vi "Begin.vi"(8 "error in":errorcluster) -> (0 "error out":errorcluster)   [LabVIEW 2020]
doc: "Called before other user functions, this VI is expected to open initial I/O refnums, load in file data, and do all program initialization. Notice that the <B>error out</B> terminal is simply used for data flow. Wiring it to other structures or subVIs ensures that this VI runs first."
uses:
  <vilib>/Rock Robotics/WPI/SafetyOutput/WPI_SafetyOutputConfigMenu.ctl
  <vilib>/Rock Robotics/WPI/DriverStation/WPI_DriverStationRobotMode2.ctl
  <vilib>/Rock Robotics/WPI/ThirdParty/REV Robotics/REVLib/Typedef/Spark MAX Motor Type.ctl
  <vilib>/Rock Robotics/WPI/ThirdParty/REV Robotics/REVLib/Typedef/Spark MAX Idle Mode.ctl
  <vilib>/Rock Robotics/WPI/ThirdParty/Phoenix-LabVIEW/Motor Controller/Controls/CTRE_Phoenix_MotorControl_ControlMode.ctl
  <vilib>/Rock Robotics/WPI/Joystick/WPI_JoystickDeviceEnum.ctl
  <vilib>/Rock Robotics/WPI/Solenoid/WPI_SolenoidChannel.ctl
  <vilib>/Rock Robotics/SystemInterfaces/i2clib/i2c_bus.ctl
  <vilib>/Rock Robotics/WPI/DriverStation/WPI_DriverStationAllianceInfo.ctl
  Robot Global Data.vi
  <vilib>/Rock Robotics/Network Tables/NT Write String Array.vi
  <vilib>/Rock Robotics/WPI/RobotDrive/WPI_RobotDriveOpen2MotorWithExistingMotors.vi
  <vilib>/Rock Robotics/WPI/Solenoid/WPI_SolenoidOpenDouble.vi
  Global Variables/StateMachineOperation.vi
panel:
  in  "Nothing":cluster{"R":dbl, "G":dbl, "B":dbl}={"R"=0.143, "G"=0.427, "B"=0.429}
  in  "Red Calibration":cluster{"R":dbl, "G":dbl, "B":dbl}={"R"=0.525, "G"=0.346, "B"=0.128}
  in  "Blue Calibration":cluster{"R":dbl, "G":dbl, "B":dbl}={"R"=0.143, "G"=0.427, "B"=0.429}
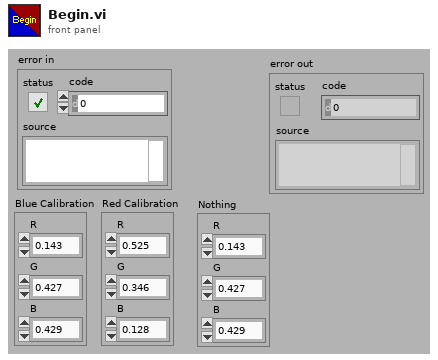
[diagram p1: front panel]
types:
  T1 = typedef "WPI_SolenoidChannel.ctl" = enum8{"Solenoid 0", "Solenoid 1", "Solenoid 2", "Solenoid 3", "Solenoid 4", "Solenoid 5", "Solenoid 6", "Solenoid 7", "Solenoid 8", "Solenoid 9", "Solenoid 10", "Solenoid 11", "Solenoid 12", "Solenoid 13", "Solenoid 14", "Solenoid 15", "Invalid"}
  T2 = typedef "WPI_DriverStationAllianceInfo.ctl" = enum16{"Red", "Blue", "Invalid"}
  T3 = typedef "i2c_bus.ctl" = enum16{"I2C On-Board", "I2C MXP", "Invalid"}
  T4 = typedef "WPI_JoystickDeviceEnum.ctl" = enum16{"USB 0", "USB 1", "USB 2", "USB 3", "USB 4", "USB 5"}
  T5 = typedef "CTRE_Phoenix_MotorControl_ControlMode.ctl" = u16
  T6 = typedef "Spark MAX Idle Mode.ctl" = enum16{"Coast", "Brake"}
  T7 = typedef "Spark MAX Motor Type.ctl" = enum16{"Brushed", "Brushless"}
  T8 = typedef "WPI_DriverStationRobotMode2.ctl" = enum16{"Autonomous Disabled", "Autonomous Enabled", "Teleop Disabled", "Teleop Enabled", "Disconnected", "Finish", "Test Disabled", "Test Enabled", "Emergency Stopped"}
  T9 = typedef "WPI_SafetyOutputConfigMenu.ctl" = enum16{"Enable", "Disable"}
  T10 = typedef "WPI_MotorControlDeviceRef.ctl" = cluster{"DeviceStatus":errorcluster, "Type":T11, "PWM":cluster{"PWM Channel":T12, "DeadBand":T13}, "CAN":cluster{"Device Number":u8, "SetOutput VI Ref":variant, "GetOutput VI Ref":variant, "Enable VI Ref":variant, "Disable VI Ref":variant, "Data":variant}, "Invert":bool, "DIO PWM":cluster{"PWM \"Enable\" Channel":T12, "DIOChannel":T14, "PWM Rate":dbl}}
  T11 = typedef "WPI_MotorControlType.ctl" = enum16{"PWM", "CAN", "DIO PWM"}
  T12 = typedef "FPGA_DIOPWMChannel.ctl" = enum8{"PWM 0", "PWM 1", "PWM 2", "PWM 3", "PWM 4", "PWM 5", "PWM 6", "PWM 7", "PWM 8", "PWM 9", "PWM MXP 0", "PWM MXP 1", "PWM MXP 2", "PWM MXP 3", "PWM MXP 4", "PWM MXP 5", "PWM MXP 6", "PWM MXP 7", "PWM MXP 8", "PWM MXP 9", "Invalid"}
  T13 = typedef "WPI_PWMDeadband.ctl" = cluster{"Name":string, "maxPositivePwm":i32, "minPositivePwm":i32, "centerPwm":i32, "maxNegativePwm":i32, "minNegativePwm":i32, "angularRange":u16}
  T14 = typedef "FPGA_DIOChannel.ctl" = enum8{"DIO 0", "DIO 1", "DIO 2", "DIO 3", "DIO 4", "DIO 5", "DIO 6", "DIO 7", "DIO 8", "DIO 9", "DIO MXP 0", "DIO MXP 1", "DIO MXP 2", "DIO MXP 3", "DIO MXP 4", "DIO MXP 5", "DIO MXP 6", "DIO MXP 7", "DIO MXP 8", "DIO MXP 9", "DIO MXP 10", "DIO MXP 11", "DIO MXP 12", "DIO MXP 13", "DIO MXP 14", "DIO MXP 15", "SPI Port CS1", "SPI Port CS2", "SPI Port CS3", "SPI Port MISO", "SPI Port MOSI", "Invalid"}
  T15 = typedef "WPI_JoystickDevRef.ctl" = cluster{"Device":T4}
  T16 = typedef "WPI_RobotDriveDevRef.ctl" = cluster{"DevStatus":errorcluster, "Motors[]":T10[], "Square Inputs":bool, "Max Output":dbl}
  T17 = typedef "WPI_SolenoidDevRef.ctl" = cluster{"DevStatus":errorcluster, "Pneumatics Control Module":u8, "Forward Solenoid Channel":T1, "Reverse Solenoid Channel":T1}
  T18 = typedef "Color Sensor V3 DevRef.ctl" = cluster{"I2CDevRef":T19}
  T19 = typedef "WPI_I2CDevRef.ctl" = cluster{"DevStatus":errorcluster, "Device Address":u8, "Handle":i32, "I2C Bus":T3}
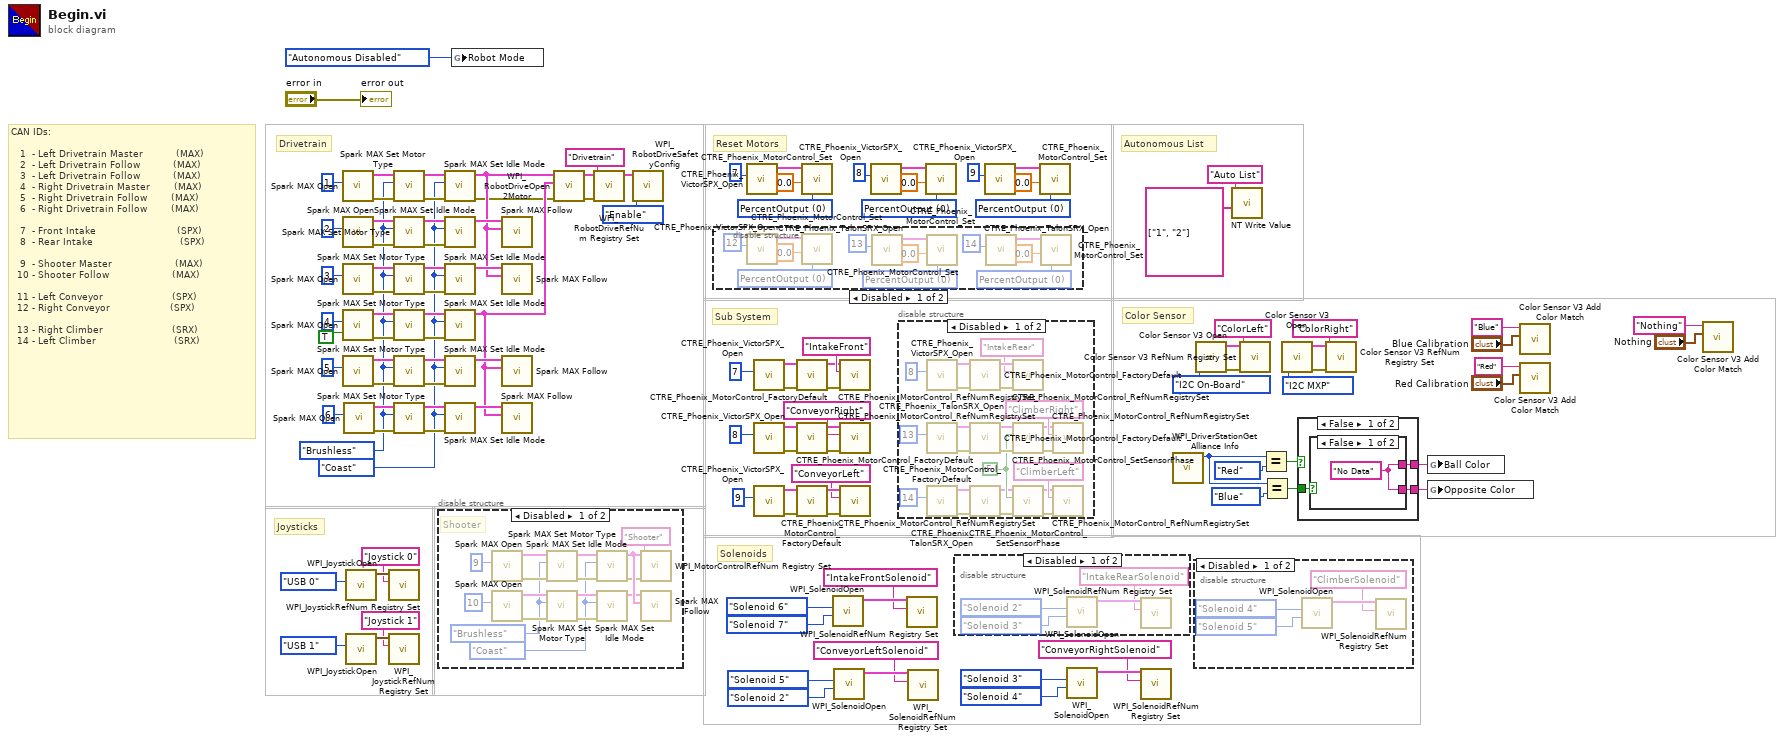
[diagram p0: block diagram]
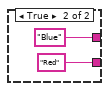
[diagram p6: hidden frame]
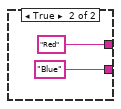
[diagram p7: hidden frame]
diagram:
  w59 = T5 0 items=["PercentOutput"=0, "Position"=1, "Velocity"=2, "Current"=3, "Follower"=5, "MotionProfile"=6, "MotionMagic"=7, "MotionProfileArc"=10, "Disabled"=15] ("Control Mode")
  w64 = T5 0 items=["PercentOutput"=0, "Position"=1, "Velocity"=2, "Current"=3, "Follower"=5, "MotionProfile"=6, "MotionMagic"=7, "MotionProfileArc"=10, "Disabled"=15] ("Control Mode")
  w68 = T5 0 items=["PercentOutput"=0, "Position"=1, "Velocity"=2, "Current"=3, "Follower"=5, "MotionProfile"=6, "MotionMagic"=7, "MotionProfileArc"=10, "Disabled"=15] ("Control Mode")
  w70 = Spark_MAX_Idle_Mode."Coast" ("Idle Mode")
  w71 = Spark_MAX_Motor_Type."Brushless" ("Motor Type")
  # "Color Sensor"
  # "Solenoids"
  # "Joysticks"
  # "Autonomous List"
  # "Sub System"
  # "CAN IDs:\n\n   1  - Left Drivetrain Master           (MAX)\n   2  - Left Drivetrain Follow           (MAX)\n   3  - Left Drivetrain Follow           (MAX)\n   4  - Right Drivetrain Master        (MAX)\n   5  - Right Drivetrain Follow        (MAX)\n   6  - Right Drivetrain Follow        (MAX)\n\n   7  - Front Intake                           (SPX)\n   8  - Rear Intake                             (SPX)\n\n   9  - Shooter Master                     (MAX)\n  10 - Shooter Follow                     (MAX)\n\n  11 - Left Conveyor                       (SPX)\n  12 - Right Conveyor                    (SPX)\n\n  13 - Right Climber                       (SRX)\n  14 - Left Climber                          (SRX)"
  # "Reset Motors"
  # "Drivetrain"
  n1 = call <vilib>:"Spark MAX Open.vi"("Device Number"=u8 1) -> ("error out"=w109:errorcluster, "MotorControlDeviceRef"=w108:T10)  [unwired: 9 in]
  n2 = call <vilib>:"Spark MAX Open.vi"("Device Number"=u8 2) -> ("error out"=w105:errorcluster, "MotorControlDeviceRef"=w104:T10)  [unwired: 9 in]
  n3 = call <vilib>:"Spark MAX Open.vi"("Device Number"=u8 3) -> ("error out"=w100:errorcluster, "MotorControlDeviceRef"=w99:T10)  [unwired: 9 in]
  n4 = call <vilib>:"Spark MAX Open.vi"("Invert"=TRUE, "Device Number"=u8 4) -> ("error out"=w95:errorcluster, "MotorControlDeviceRef"=w94:T10)  [unwired: 8 in]
  n5 = call <vilib>:"Spark MAX Open.vi"("Device Number"=u8 5) -> ("error out"=w91:errorcluster, "MotorControlDeviceRef"=w90:T10)  [unwired: 9 in]
  n6 = call <vilib>:"Spark MAX Open.vi"("Device Number"=u8 6) -> ("error out"=w86:errorcluster, "MotorControlDeviceRef"=w85:T10)  [unwired: 9 in]
  n7 = call <vilib>:"WPI_JoystickOpen.vi"("JoystickDevice"=WPI_JoystickDeviceEnum."USB 0") -> ("JoystickDevRef"=w38:T15)  [unwired: 10 in]
  n8 = call <vilib>:"WPI_JoystickOpen.vi"("JoystickDevice"=WPI_JoystickDeviceEnum."USB 1") -> ("JoystickDevRef"=w35:T15)  [unwired: 10 in]
  n9 = call <vilib>:"WPI_JoystickRefNum Registry Set.vi"("refnum name"="Joystick 0", "JoystickDevRef"=w38) -> ()  [unwired: 8 in, 2 out]
  n10 = call <vilib>:"WPI_JoystickRefNum Registry Set.vi"("refnum name"="Joystick 1", "JoystickDevRef"=w35) -> ()  [unwired: 8 in, 2 out]
  n11 = call <vilib>:"Spark MAX Set Motor Type.vi"("error in (no error)"=w109, "Motor Type"=w71, "MotorControlDevRef"=w108) -> ("error out"=w107:errorcluster, "MotorControlDeviceRef"=w106:T10)  [unwired: 7 in]
  n12 = call <vilib>:"Spark MAX Set Motor Type.vi"("error in (no error)"=w105, "Motor Type"=w71, "MotorControlDevRef"=w104) -> ("error out"=w103:errorcluster, "MotorControlDeviceRef"=w102:T10)  [unwired: 7 in]
  n13 = call <vilib>:"Spark MAX Set Motor Type.vi"("error in (no error)"=w100, "Motor Type"=w71, "MotorControlDevRef"=w99) -> ("error out"=w98:errorcluster, "MotorControlDeviceRef"=w97:T10)  [unwired: 7 in]
  n14 = call <vilib>:"Spark MAX Set Motor Type.vi"("error in (no error)"=w95, "Motor Type"=w71, "MotorControlDevRef"=w94) -> ("error out"=w93:errorcluster, "MotorControlDeviceRef"=w92:T10)  [unwired: 7 in]
  n15 = call <vilib>:"Spark MAX Set Motor Type.vi"("error in (no error)"=w91, "Motor Type"=w71, "MotorControlDevRef"=w90) -> ("error out"=w89:errorcluster, "MotorControlDeviceRef"=w88:T10)  [unwired: 7 in]
  n16 = call <vilib>:"Spark MAX Set Motor Type.vi"("error in (no error)"=w86, "Motor Type"=w71, "MotorControlDevRef"=w85) -> ("error out"=w84:errorcluster, "MotorControlDeviceRef"=w83:T10)  [unwired: 7 in]
  n17 = disable-structure shown="Disabled" {
    frame Disabled {
      w123 = Spark_MAX_Idle_Mode."Coast" ("Idle Mode")
      w124 = Spark_MAX_Motor_Type."Brushless" ("Motor Type")
      # "Shooter"
      n18 = call <vilib>:"Spark MAX Open.vi"("Device Number"=u8 9) -> ("error out"=w134:errorcluster, "MotorControlDeviceRef"=w133:T10)  [unwired: 9 in]
      n19 = call <vilib>:"Spark MAX Open.vi"("Device Number"=u8 10) -> ("error out"=w128:errorcluster, "MotorControlDeviceRef"=w131:T10)  [unwired: 9 in]
      n20 = call <vilib>:"Spark MAX Set Motor Type.vi"("error in (no error)"=w134, "Motor Type"=w124, "MotorControlDevRef"=w133) -> ("error out"=w127:errorcluster, "MotorControlDeviceRef"=w122:T10)  [unwired: 7 in]
      n21 = call <vilib>:"Spark MAX Set Motor Type.vi"("error in (no error)"=w128, "Motor Type"=w124, "MotorControlDevRef"=w131) -> ("error out"=w125:errorcluster, "MotorControlDeviceRef"=w130:T10)  [unwired: 7 in]
      n22 = call <vilib>:"Spark MAX Set Idle Mode.vi"("error in (no error)"=w127, "Idle Mode"=w123, "MotorControlDeviceRef in"=w122) -> ("error out"=w126:errorcluster, "MotorControlDeviceRef out"=w132:T10)  [unwired: 7 in]
      n23 = call <vilib>:"Spark MAX Set Idle Mode.vi"("error in (no error)"=w125, "Idle Mode"=w123, "MotorControlDeviceRef in"=w130) -> ("MotorControlDeviceRef out"=w129:T10)  [unwired: 7 in, 1 out]
      n24 = call <vilib>:"WPI_MotorControlRefNum Registry Set.vi"("error in (no error)"=w126, "refnum name"="Shooter", "MotorControlDevRef"=w132) -> ()  [unwired: 7 in, 2 out]
      n25 = call <vilib>:"Spark MAX Follow.vi"("Master Controller"=w132, "MotorControlDeviceRef"=w129) -> ()  [unwired: 8 in, 2 out]
    }
    frame Enabled {
    }
  }
  n26 = call <vilib>:"Spark MAX Set Idle Mode.vi"("error in (no error)"=w107, "Idle Mode"=w70, "MotorControlDeviceRef in"=w106) -> ("error out"=w72:errorcluster, "MotorControlDeviceRef out"=w74:T10)  [unwired: 7 in]
  n27 = call <vilib>:"Spark MAX Set Idle Mode.vi"("error in (no error)"=w103, "Idle Mode"=w70, "MotorControlDeviceRef in"=w102) -> ("MotorControlDeviceRef out"=w101:T10)  [unwired: 7 in, 1 out]
  n28 = call <vilib>:"Spark MAX Set Idle Mode.vi"("error in (no error)"=w98, "Idle Mode"=w70, "MotorControlDeviceRef in"=w97) -> ("MotorControlDeviceRef out"=w96:T10)  [unwired: 7 in, 1 out]
  n29 = call <vilib>:"Spark MAX Set Idle Mode.vi"("error in (no error)"=w93, "Idle Mode"=w70, "MotorControlDeviceRef in"=w92) -> ("MotorControlDeviceRef out"=w73:T10)  [unwired: 7 in, 1 out]
  n30 = call <vilib>:"Spark MAX Set Idle Mode.vi"("error in (no error)"=w89, "Idle Mode"=w70, "MotorControlDeviceRef in"=w88) -> ("MotorControlDeviceRef out"=w87:T10)  [unwired: 7 in, 1 out]
  n31 = call <vilib>:"Spark MAX Set Idle Mode.vi"("error in (no error)"=w84, "Idle Mode"=w70, "MotorControlDeviceRef in"=w83) -> ("MotorControlDeviceRef out"=w82:T10)  [unwired: 7 in, 1 out]
  n32 = global write "Robot Global Data.vi" "Robot Mode"(WPI_DriverStationRobotMode2."Autonomous Disabled" ("Robot Mode")) -> ()
  n33 = call <vilib>:"Spark MAX Follow.vi"("Master Controller"=w74, "MotorControlDeviceRef"=w101) -> ()  [unwired: 8 in, 2 out]
  n34 = call <vilib>:"Spark MAX Follow.vi"("Master Controller"=w74, "MotorControlDeviceRef"=w96) -> ()  [unwired: 8 in, 2 out]
  n35 = call <vilib>:"Spark MAX Follow.vi"("Master Controller"=w73, "MotorControlDeviceRef"=w87) -> ()  [unwired: 8 in, 2 out]
  n36 = call <vilib>:"Spark MAX Follow.vi"("Master Controller"=w73, "MotorControlDeviceRef"=w82) -> ()  [unwired: 8 in, 2 out]
  n37 = call-poly <vilib>:"WPI_RobotDriveOpen2Motor.vi"("error in (no error)"=w72, "Right Motor Dev Ref"=w73, "Left Motor Dev Ref"=w74) -> ("error out"=w116:errorcluster, "RobotDriveDevRef"=w118:T16)  [unwired: 2 in, 5 out]
  n38 = call <vilib>:"WPI_RobotDriveRefNum Registry Set.vi"("error in (no error)"=w116, "refnum name"="Drivetrain", "RobotDriveDevRef"=w118) -> ("RobotDriveDevRef"=w115:T16)  [unwired: 1 in, 7 out]
  n39 = call <vilib>:"WPI_RobotDriveSafetyConfig.vi"("mode"=WPI_SafetyOutputConfigMenu."Enable", "RobotDriveDevRef"=w115) -> ()  [unwired: 8 in, 2 out]
  n40 = disable-structure shown="Disabled" {
    frame Disabled {
      w136 = T5 0 items=["PercentOutput"=0, "Position"=1, "Velocity"=2, "Current"=3, "Follower"=5, "MotionProfile"=6, "MotionMagic"=7, "MotionProfileArc"=10, "Disabled"=15] ("Control Mode")
      w141 = T5 0 items=["PercentOutput"=0, "Position"=1, "Velocity"=2, "Current"=3, "Follower"=5, "MotionProfile"=6, "MotionMagic"=7, "MotionProfileArc"=10, "Disabled"=15] ("Control Mode")
      w144 = T5 0 items=["PercentOutput"=0, "Position"=1, "Velocity"=2, "Current"=3, "Follower"=5, "MotionProfile"=6, "MotionMagic"=7, "MotionProfileArc"=10, "Disabled"=15] ("Control Mode")
      n41 = call <vilib>:"CTRE_Phoenix_VictorSPX_Open.vi"("Device Number"=u8 12) -> ("PhoenixMotorControlDevRef"=w145:T10)  [unwired: 9 in, 1 out]
      n42 = call <vilib>:"CTRE_Phoenix_MotorControl_Set.vi"("Output"=0.0, "Control Mode"=w144, "PhoenixMotorControlDevRef"=w145) -> ()  [unwired: 7 in, 2 out]
      n43 = call <vilib>:"CTRE_Phoenix_TalonSRX_Open.vi"("Device Number"=u8 13) -> ("PhoenixMotorControlDevRef"=w139:T10)  [unwired: 9 in, 1 out]
      n44 = call <vilib>:"CTRE_Phoenix_MotorControl_Set.vi"("Output"=0.0, "Control Mode"=w141, "PhoenixMotorControlDevRef"=w139) -> ()  [unwired: 7 in, 2 out]
      n45 = call <vilib>:"CTRE_Phoenix_TalonSRX_Open.vi"("Device Number"=u8 14) -> ("PhoenixMotorControlDevRef"=w138:T10)  [unwired: 9 in, 1 out]
      n46 = call <vilib>:"CTRE_Phoenix_MotorControl_Set.vi"("Output"=0.0, "Control Mode"=w136, "PhoenixMotorControlDevRef"=w138) -> ()  [unwired: 7 in, 2 out]
    }
    frame Enabled {
    }
  }
  n47 = call <vilib>:"CTRE_Phoenix_VictorSPX_Open.vi"("Device Number"=u8 7) -> ("PhoenixMotorControlDevRef"=w67:T10)  [unwired: 9 in, 1 out]
  n48 = call <vilib>:"CTRE_Phoenix_VictorSPX_Open.vi"("Device Number"=u8 7) -> ("error out"=w53:errorcluster, "PhoenixMotorControlDevRef"=w56:T10)  [unwired: 9 in]
  n49 = call <vilib>:"CTRE_Phoenix_VictorSPX_Open.vi"("Device Number"=u8 8) -> ("error out"=w50:errorcluster, "PhoenixMotorControlDevRef"=w47:T10)  [unwired: 9 in]
  n50 = call <vilib>:"CTRE_Phoenix_VictorSPX_Open.vi"("Device Number"=u8 9) -> ("error out"=w44:errorcluster, "PhoenixMotorControlDevRef"=w41:T10)  [unwired: 9 in]
  n51 = call <vilib>:"CTRE_Phoenix_MotorControl_FactoryDefault.vi"("error in"=w53, "PhoenixMotorControlDevRef"=w56) -> ("error out"=w52:errorcluster, "PhoenixMotorControlDevRef"=w54:T10)  [unwired: 8 in]
  n52 = call <vilib>:"CTRE_Phoenix_MotorControl_FactoryDefault.vi"("error in"=w50, "PhoenixMotorControlDevRef"=w47) -> ("error out"=w51:errorcluster, "PhoenixMotorControlDevRef"=w49:T10)  [unwired: 8 in]
  n53 = call <vilib>:"CTRE_Phoenix_MotorControl_FactoryDefault.vi"("error in"=w44, "PhoenixMotorControlDevRef"=w41) -> ("error out"=w45:errorcluster, "PhoenixMotorControlDevRef"=w43:T10)  [unwired: 8 in]
  n54 = call <vilib>:"CTRE_Phoenix_MotorControl_Set.vi"("Output"=0.0, "Control Mode"=w68, "PhoenixMotorControlDevRef"=w67) -> ()  [unwired: 7 in, 2 out]
  n55 = call-poly <vilib>:"WPI_SolenoidOpen.vi"("Reverse Solenoid Channel"=WPI_SolenoidChannel."Solenoid 7", "Forward Solenoid Channel"=WPI_SolenoidChannel."Solenoid 6") -> ("SolenoidDevRef"=w33:T17)  [unwired: 8 in, 1 out]
  n56 = call-poly <vilib>:"WPI_SolenoidOpen.vi"("Reverse Solenoid Channel"=WPI_SolenoidChannel."Solenoid 2", "Forward Solenoid Channel"=WPI_SolenoidChannel."Solenoid 5") -> ("SolenoidDevRef"=w10:T17)  [unwired: 8 in, 1 out]
  n57 = call <vilib>:"CTRE_Phoenix_MotorControl_RefNumRegistrySet.vi"("error in (no error)"=w52, "refnum name"="IntakeFront", "PhoenixMotorControlDevRef"=w54) -> ()  [unwired: 7 in, 2 out]
  n58 = call <vilib>:"CTRE_Phoenix_MotorControl_RefNumRegistrySet.vi"("error in (no error)"=w51, "refnum name"="ConveyorRight", "PhoenixMotorControlDevRef"=w49) -> ()  [unwired: 7 in, 2 out]
  n59 = call <vilib>:"CTRE_Phoenix_MotorControl_RefNumRegistrySet.vi"("error in (no error)"=w45, "refnum name"="ConveyorLeft", "PhoenixMotorControlDevRef"=w43) -> ()  [unwired: 7 in, 2 out]
  n60 = call <vilib>:"CTRE_Phoenix_VictorSPX_Open.vi"("Device Number"=u8 8) -> ("PhoenixMotorControlDevRef"=w62:T10)  [unwired: 9 in, 1 out]
  n61 = disable-structure shown="Disabled" {
    frame Disabled {
      w155 = FALSE ("PhaseSensor")
      n62 = call <vilib>:"CTRE_Phoenix_VictorSPX_Open.vi"("Device Number"=u8 8) -> ("error out"=w168:errorcluster, "PhoenixMotorControlDevRef"=w165:T10)  [unwired: 9 in]
      n63 = call <vilib>:"CTRE_Phoenix_TalonSRX_Open.vi"("Device Number"=u8 13) -> ("error out"=w162:errorcluster, "PhoenixMotorControlDevRef"=w163:T10)  [unwired: 9 in]
      n64 = call <vilib>:"CTRE_Phoenix_TalonSRX_Open.vi"("Device Number"=u8 14) -> ("error out"=w160:errorcluster, "PhoenixMotorControlDevRef"=w161:T10)  [unwired: 9 in]
      n65 = call <vilib>:"CTRE_Phoenix_MotorControl_FactoryDefault.vi"("error in"=w168, "PhoenixMotorControlDevRef"=w165) -> ("error out"=w169:errorcluster, "PhoenixMotorControlDevRef"=w167:T10)  [unwired: 8 in]
      n66 = call <vilib>:"CTRE_Phoenix_MotorControl_FactoryDefault.vi"("error in"=w162, "PhoenixMotorControlDevRef"=w163) -> ("error out"=w156:errorcluster, "PhoenixMotorControlDevRef"=w157:T10)  [unwired: 8 in]
      n67 = call <vilib>:"CTRE_Phoenix_MotorControl_FactoryDefault.vi"("error in"=w160, "PhoenixMotorControlDevRef"=w161) -> ("error out"=w154:errorcluster, "PhoenixMotorControlDevRef"=w152:T10)  [unwired: 8 in]
      n68 = call <vilib>:"CTRE_Phoenix_MotorControl_RefNumRegistrySet.vi"("error in (no error)"=w169, "refnum name"="IntakeRear", "PhoenixMotorControlDevRef"=w167) -> ()  [unwired: 7 in, 2 out]
      n69 = call <vilib>:"CTRE_Phoenix_MotorControl_SetSensorPhase.vi"("error in (no error)"=w156, "PhaseSensor"=w155, "PhoenixMotorControlDevRef"=w157) -> ("error out"=w147:errorcluster, "PhoenixMotorControlDevRef"=w150:T10)  [unwired: 7 in]
      n70 = call <vilib>:"CTRE_Phoenix_MotorControl_SetSensorPhase.vi"("error in (no error)"=w154, "PhaseSensor"=w155, "PhoenixMotorControlDevRef"=w152) -> ("error out"=w153:errorcluster, "PhoenixMotorControlDevRef"=w151:T10)  [unwired: 7 in]
      n71 = call <vilib>:"CTRE_Phoenix_MotorControl_RefNumRegistrySet.vi"("error in (no error)"=w147, "refnum name"="ClimberRight", "PhoenixMotorControlDevRef"=w150) -> ()  [unwired: 7 in, 2 out]
      n72 = call <vilib>:"CTRE_Phoenix_MotorControl_RefNumRegistrySet.vi"("error in (no error)"=w153, "refnum name"="ClimberLeft", "PhoenixMotorControlDevRef"=w151) -> ()  [unwired: 7 in, 2 out]
    }
    frame Enabled {
    }
  }
  n73 = call <vilib>:"WPI_SolenoidRefNum Registry Set.vi"("refnum name"="IntakeFrontSolenoid", "SolenoidDevRef"=w33) -> ()  [unwired: 8 in, 2 out]
  n74 = call <vilib>:"WPI_SolenoidRefNum Registry Set.vi"("refnum name"="ConveyorLeftSolenoid", "SolenoidDevRef"=w10) -> ()  [unwired: 8 in, 2 out]
  n75 = call <vilib>:"CTRE_Phoenix_MotorControl_Set.vi"("Output"=0.0, "Control Mode"=w64, "PhoenixMotorControlDevRef"=w62) -> ()  [unwired: 7 in, 2 out]
  n76 = disable-structure shown="Disabled" {
    frame Disabled {
      n77 = call-poly <vilib>:"WPI_SolenoidOpen.vi"("Reverse Solenoid Channel"=WPI_SolenoidChannel."Solenoid 3", "Forward Solenoid Channel"=WPI_SolenoidChannel."Solenoid 2") -> ("SolenoidDevRef"=w173:T17)  [unwired: 8 in, 1 out]
      n78 = call <vilib>:"WPI_SolenoidRefNum Registry Set.vi"("refnum name"="IntakeRearSolenoid", "SolenoidDevRef"=w173) -> ()  [unwired: 8 in, 2 out]
    }
    frame Enabled {
    }
  }
  n79 = call <vilib>:"CTRE_Phoenix_VictorSPX_Open.vi"("Device Number"=u8 9) -> ("PhoenixMotorControlDevRef"=w61:T10)  [unwired: 9 in, 1 out]
  n80 = call <vilib>:"CTRE_Phoenix_MotorControl_Set.vi"("Output"=0.0, "Control Mode"=w59, "PhoenixMotorControlDevRef"=w61) -> ()  [unwired: 7 in, 2 out]
  n81 = call-poly <vilib>:"WPI_SolenoidOpen.vi"("Reverse Solenoid Channel"=WPI_SolenoidChannel."Solenoid 4", "Forward Solenoid Channel"=WPI_SolenoidChannel."Solenoid 3") -> ("SolenoidDevRef"=w6:T17)  [unwired: 8 in, 1 out]
  n82 = call <vilib>:"WPI_SolenoidRefNum Registry Set.vi"("refnum name"="ConveyorRightSolenoid", "SolenoidDevRef"=w6) -> ()  [unwired: 8 in, 2 out]
  n83 = call <vilib>:"WPI_DriverStationGet Alliance Info.vi"() -> ("Alliance"=w17:T2)  [unwired: 6 in, 5 out]
  n84 = disable-structure shown="Disabled" {
    frame Disabled {
      n85 = call-poly <vilib>:"WPI_SolenoidOpen.vi"("Reverse Solenoid Channel"=WPI_SolenoidChannel."Solenoid 5", "Forward Solenoid Channel"=WPI_SolenoidChannel."Solenoid 4") -> ("SolenoidDevRef"=w177:T17)  [unwired: 8 in, 1 out]
      n86 = call <vilib>:"WPI_SolenoidRefNum Registry Set.vi"("refnum name"="ClimberSolenoid", "SolenoidDevRef"=w177) -> ()  [unwired: 8 in, 2 out]
    }
    frame Enabled {
    }
  }
  n87 = call <vilib>:"Color Sensor V3 Open.vi"("I2C Bus"=i2c_bus."I2C On-Board") -> ("error out"=w23:errorcluster, "ColorSensorDevRef"=w21:T18)  [unwired: 9 in]
  n88 = call-poly <vilib>:"NT Write Value.vi"("String Array"=string[] ["1", "2"], "Name"="Auto List") -> ()  [unwired: 9 in, 1 out]
  n89 = call <vilib>:"Color Sensor V3 RefNum Registry Set.vi"("error in (no error)"=w23, "refnum name"="ColorLeft", "ColorSensorDevRef"=w21) -> ()  [unwired: 7 in, 2 out]
  n90 = Equal?(x=w17, y=WPI_DriverStationAllianceInfo."Red") -> (x = y?=w14:bool)
  n91 = Equal?(x=w17, y=WPI_DriverStationAllianceInfo."Blue") -> (x = y?=w11:bool)
  n92 = call <vilib>:"Color Sensor V3 Open.vi"("I2C Bus"=i2c_bus."I2C MXP") -> ("error out"=w24:errorcluster, "ColorSensorDevRef"=w29:T18)  [unwired: 9 in]
  n93 = case shown="False" w14 {
    tunnel: [w179 "Red"] -> w13
    tunnel: [w178 "Blue"] -> w12
    tunnel: w11 -> [w180 _]
    frame False {
      n94 = case shown="False" w180 {
        tunnel: [w181 "Blue"] -> w179
        tunnel: [w181 "Red"] -> w178
        frame False {
          w181 = "No Data"
        }
        frame True {
        }
      }
    }
    frame True {
    }
  }
  n95 = call <vilib>:"Color Sensor V3 RefNum Registry Set.vi"("error in (no error)"=w24, "refnum name"="ColorRight", "ColorSensorDevRef"=w29) -> ()  [unwired: 7 in, 2 out]
  n96 = global write "StateMachineOperation.vi" "Ball Color"(w13) -> ()
  n97 = global write "StateMachineOperation.vi" "Opposite Color"(w12) -> ()
  n98 = call <vilib>:"Color Sensor V3 Add Color Match.vi"("Color"="Blue Calibration", "Name"="Blue") -> ()  [unwired: 10 in]
  n99 = call <vilib>:"Color Sensor V3 Add Color Match.vi"("Color"="Red Calibration", "Name"="Red") -> ()  [unwired: 10 in]
  n100 = call <vilib>:"Color Sensor V3 Add Color Match.vi"("Color"="Nothing", "Name"="Nothing") -> ()  [unwired: 10 in]
  "error out" <- "error in"
